vi "Requests.vi"(8 "error in (no error)":errorcluster, 9 "write enable":bool=TRUE, 11 "ICPCON ET-7018 in":refnum<class "ICPCON ET-7018.lvclass">) -> (0 "error out":errorcluster, 3 "ICPCON ET-7018 out":refnum<class "ICPCON ET-7018.lvclass">)   [LabVIEW 2019, in "ICPCON ET-7018.lvclass"]
uses:
  ICPCON ET-7018.lvclass
  D:/my_projects/projects/Algorithms/Labview/19/Modbus/MB_TCP2/MB_TCP.lvclass
  MB_TCP.lvclass/MB_TCP.ctl
  NI_modbus_upd/Ctl/Unit_ID.ctl
  NI_modbus_upd/TCP/TCP.lvclass/TCP.ctl
  NI_modbus_upd/Function data mismatch error1.vi
  NI_modbus_upd/Master Function Definition/Responses/Write Multiple Coils Response.vi
  NI_modbus_upd/Master network read write.vi
  NI_modbus_upd/Master Function Definition/Requests/Write Multiple Coils Request.vi
  NI_modbus_upd/Master Function Definition/Responses/Read Coils Response.vi
  NI_modbus_upd/Master Function Definition/Requests/Read Coils Request.vi
  NI_modbus_upd/Master Function Definition/Responses/Read Input Registers Response.vi
  NI_modbus_upd/Master Function Definition/Requests/Read Input Registers Request.vi
  NI_modbus_upd/Error Generator1.vi
  NI_modbus_upd/Function code mismatch error1.vi
  NI_modbus_upd/Read ADU Packet Master.vi
  NI_modbus_upd/Write ADU Packet Master.vi
  NI_modbus_upd/Modbus Data Unit (PDU)/Construct PDU1.vi
  NI_modbus_upd/Utility/Bits to Bytes1.vi
  NI_modbus_upd/Utility/Bytes to Bits1.vi
  NI_modbus_upd/Utility/Bytes to U16s1.vi
  NI_modbus_upd/Modbus Data Unit (PDU)/Unflatten to PDU1.vi
  NI_modbus_upd/TCP/Protocol Read.vi
  NI_modbus_upd/TCP/Protocol Write.vi
  <vilib>/Utility/error.llb/Clear Errors.vi
  NI_modbus_upd/Modbus Data Unit (PDU)/Deconstruct PDU1.vi
  NI_modbus_upd/TCP/TCP.lvclass
  ICPCON Registers/ICPCON Registers.lvlib
  MB_TCP.lvclass
  NI_modbus_upd/NI_modbus_upd.lvlib
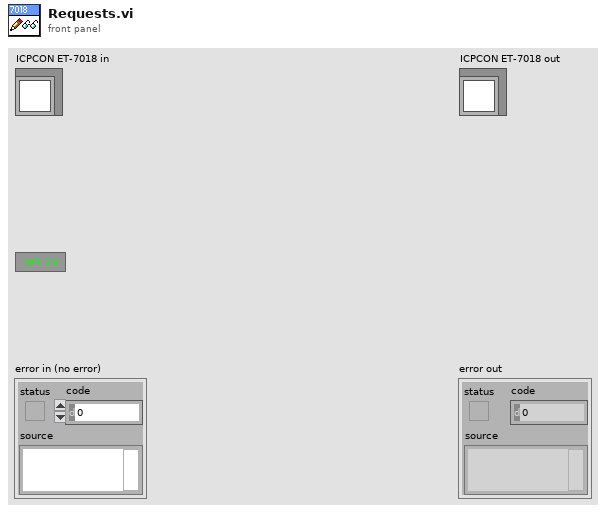
[diagram p1: front panel]
types:
  T1 = typedef "NI_modbus_upd.lvlib/Unit_ID.ctl" = cluster{"Protocol ID":u16, "Unit ID":u8}
  T2 = typedef "ICPCON Registers.lvlib/ICPCON Data.ctl" = cluster{"UTF":refnum<data-value>, "DI":refnum<data-value>, "DW":refnum<data-value>, "DO":refnum<data-value>, "IR":refnum<data-value>, "WR":refnum<data-value>, "OR":refnum<data-value>, "modified":refnum<data-value>}
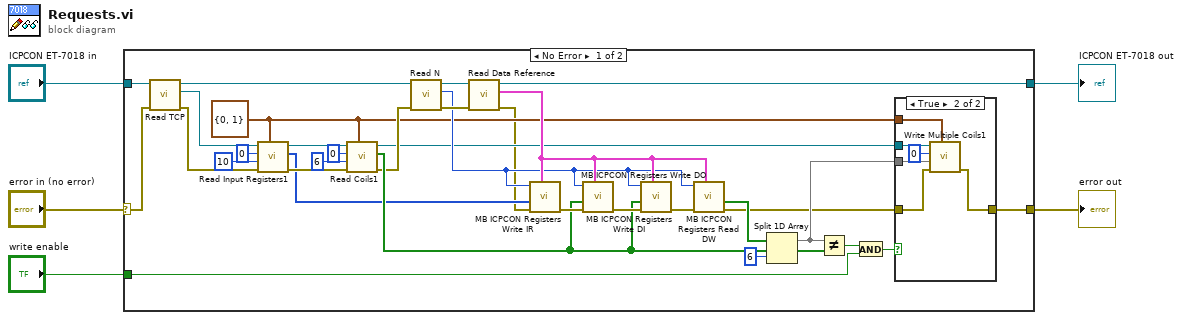
[diagram p0: block diagram]
diagram:
  n1 = case shown="No Error" "error in (no error)" {
    selector: "error in (no error)" -> [w21 w47]
    tunnel: [w26 w47] -> w3
    tunnel: [w22 w46] -> w4
    tunnel: "ICPCON ET-7018 in" -> [w24 w46]
    tunnel: "write enable" -> [w25 _]
    frame No Error {
      w7 = T1 {"Protocol ID"=0, "Unit ID"=1} ("Unit_ID")
      n2 = call "Read TCP.vi"("error in (no error)"=w21, "MB_TCP in"=w24) -> ("error out"=w17:errorcluster, "TCP"=w20:refnum<class "TCP.lvclass">, "MB_TCP out"=w23:refnum<class "ICPCON ET-7018.lvclass">)  [unwired: 7 in]
      n3 = call "Read Input Registers1.vi"("Unit_ID"=w7, "error in (no error)"=w17, "number of input registers"=u16 10, "starting address"=u16 0, "Modbus master in"=w20) -> ("error out"=w15:errorcluster, "register values"=w9:u16[], "Modbus master out"=w16:refnum<class "TCP.lvclass">)  [unwired: 4 in]
      n4 = call "Read Coils1.vi"("Unit_ID"=w7, "error in (no error)"=w15, "number of coils"=u16 6 ("number of input registers"), "starting address"=u16 0, "Modbus master in"=w16) -> ("error out"=w11:errorcluster, "coil values"=w12:bool[], "Modbus master out"=w8:refnum<class "TCP.lvclass">)  [unwired: 4 in]
      n5 = call "Read N.vi"("error in (no error)"=w11, "MB_TCP in"=w23) -> ("error out"=w38:errorcluster, "N"=w10:i32, "MB_TCP out"=w37:refnum<class "ICPCON ET-7018.lvclass">)  [unwired: 7 in]
      n6 = call "Read Data Reference.vi"("error in (no error)"=w38, "MB_TCP in"=w37) -> ("error out"=w6:errorcluster, "Data"=w27:T2, "MB_TCP out"=w22:refnum<class "ICPCON ET-7018.lvclass">)  [unwired: 7 in]
      n7 = call "MB ICPCON Registers Write IR.vi"("Data Reference"=w27, "error in (no error)"=w6, "Words In"=w9, "N"=w10) -> ("error out"=w36:errorcluster)  [unwired: 7 in]
      n8 = call "MB ICPCON Registers Write DO.vi"("Data Reference"=w27, "error in (no error)"=w36, "Bits In"=w12, "N"=w10) -> ("error out"=w35:errorcluster)  [unwired: 7 in]
      n9 = call "MB ICPCON Registers Write DI.vi"("Data Reference"=w27, "error in (no error)"=w35, "Bits In"=w12, "N"=w10) -> ("error out"=w28:errorcluster)  [unwired: 7 in]
      n10 = call "MB ICPCON Registers Read DW.vi"("Data Reference"=w27, "error in (no error)"=w28, "N"=w10) -> ("error out"=w29:errorcluster, "Bits out"=w32:bool[])  [unwired: 7 in]
      n11 = Split 1D Array(array=w32, index=6 ("length")) -> (first subarray=w30:bool[])  [unwired: 1 out]
      n12 = Not Equal?(x=w30, y=w12) -> (x != y?=w34:bool)
      n13 = And(x=w34, y=w25) -> (x .and. y?=w33:bool)
      n14 = case shown="True" w33 {
        tunnel: w29 -> [w39 w42]
        tunnel: [w39 w40] -> w26
        tunnel: w30 -> [_ w43]
        tunnel: w8 -> [_ w45]
        tunnel: w7 -> [_ w44]
        frame False {
        }
        frame True {
          n15 = call "Write Multiple Coils1.vi"("Unit_ID"=w44, "error in (no error)"=w42, "coil values"=w43, "starting address"=u16 0, "Modbus master in"=w45) -> ("error out"=w40:errorcluster)  [unwired: 5 in, 1 out]
        }
      }
    }
    frame Error {
    }
  }
  "error out" <- w3
  "ICPCON ET-7018 out" <- w4
